vi "Show Raw Image (SubVI).vi"(0 "Display Data":T3, 5 "Image Size":T1={"Height"=512, "Width"=512} {"Width" step=8; "Height" step=8}) -> (14 "Image Out":T2)   [LabVIEW 2017]
uses:
  Controls (HOST)/Image Size.ctl
  Controls (HOST)/Data to Disk Bundle.ctl
  <vilib>/vision/Image Controls.llb/IMAQ Image.ctl
panel:
  in  "Image Size 2":T1={"Height"=512, "Width"=512} {"Width" step=8; "Height" step=8}
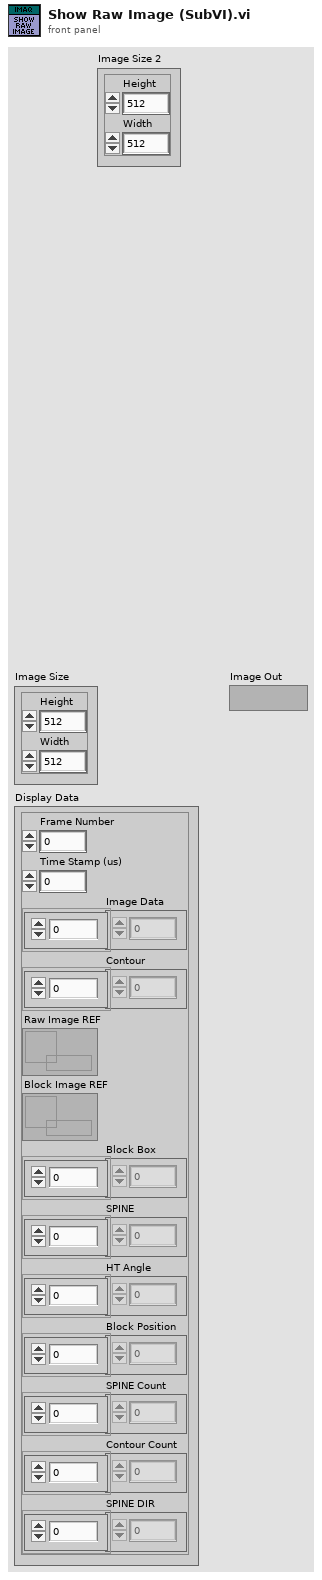
[diagram p1: front panel]
types:
  T1 = typedef "Image Size.ctl" = cluster{"Height":u16, "Width":u16}
  T2 = typedef "IMAQ Image.ctl" = refnum<image>
  T3 = typedef "Data to Disk Bundle.ctl" = cluster{"Frame Number":u64, "Time Stamp (us)":u64, "Image Data":u64[], "Contour":u32[], "Raw Image REF":refnum<data-value>, "Block Image REF":refnum<data-value>, "Block Box":u64[], "SPINE":u32[], "HT Angle":u64[], "Block Position":u64[], "SPINE Count":u32[], "Contour Count":u32[], "SPINE DIR":u8[]}
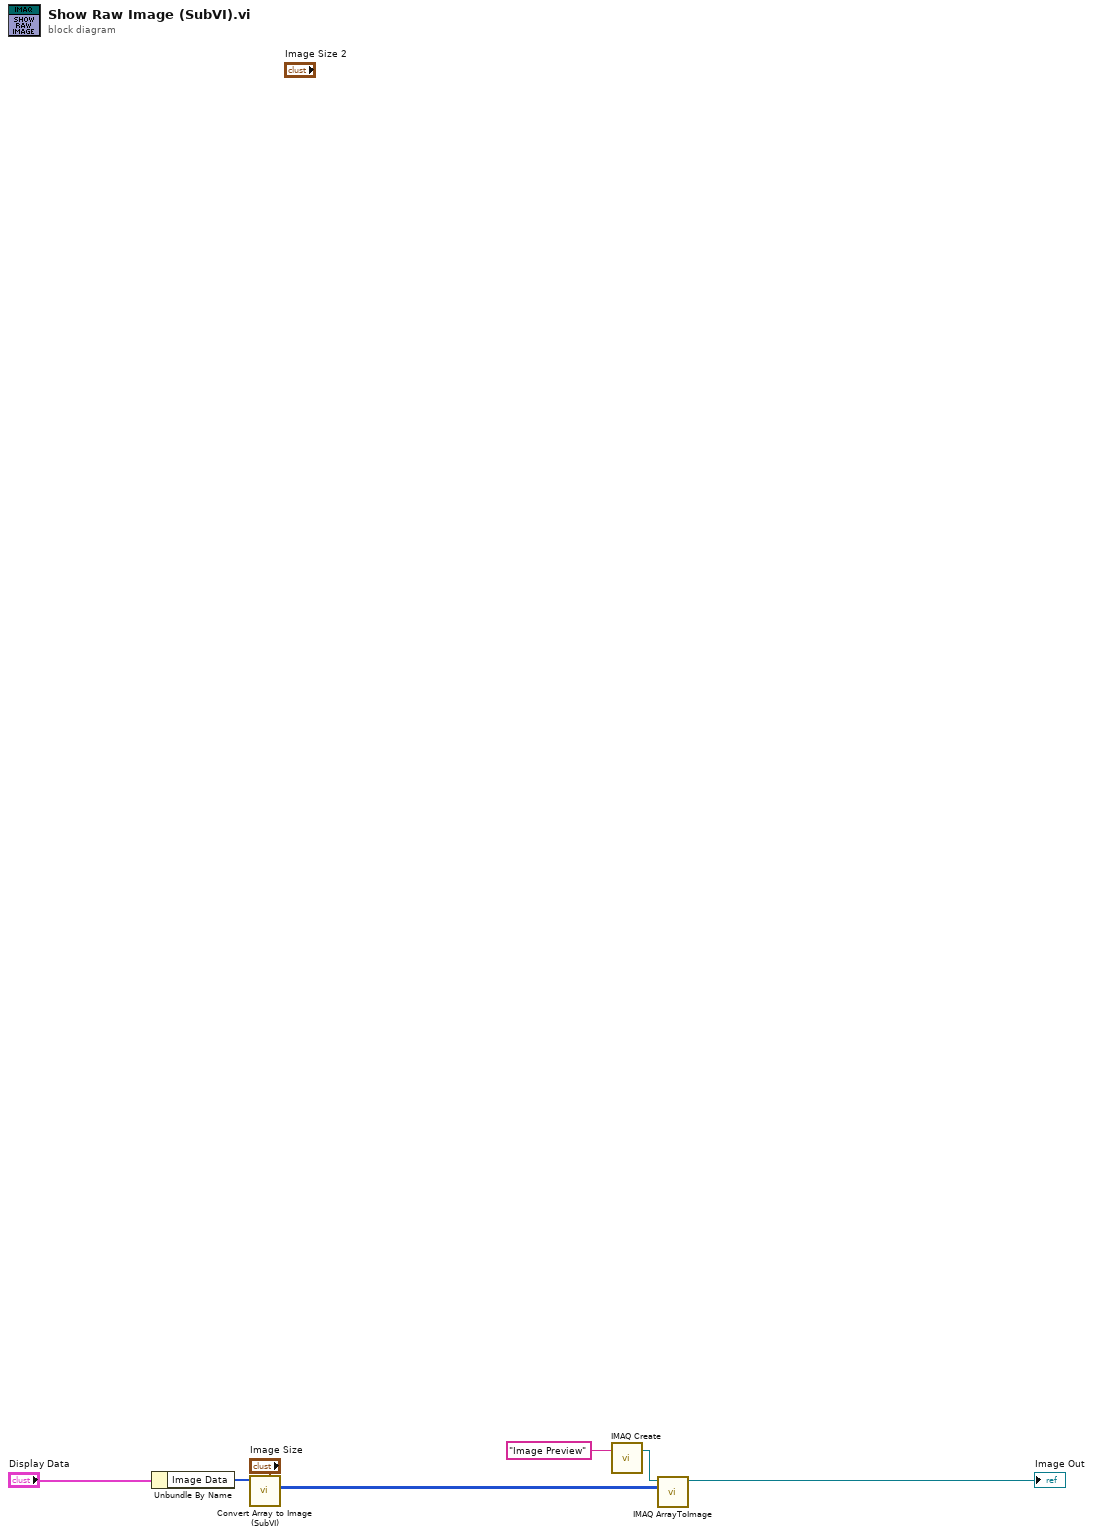
[diagram p0: block diagram]
diagram:
  n1 = Unbundle By Name("Display Data") -> ("Image Data"=w5:u64[])
  n2 = call "Convert Array to Image (SubVI).vi"("Image Size"="Image Size", "Image Array In"=w5) -> ("Image Array Out"=w3:u8[][])  [unwired: 9 in]
  n3 = call "IMAQ Create"("Image Name"="Image Preview") -> ("New Image"=w4:T2)  [unwired: 4 in, 1 out]
  n4 = call "IMAQ ArrayToImage"("Image Pixels (U8)"=w3, "Image"=w4) -> ("Image Out"=→"Image Out":T2)  [unwired: 8 in, 1 out]
